vi "File et notification.vi"(8 "error in (no error)":errorcluster caption="entrée d'erreur (pas d'erreur)") -> (0 "error out":errorcluster caption="sortie d'erreur", 3 "File et Queue":T2)   [LabVIEW 2020]
uses:
  File et notification.ctl
  TypeDef/Data Event Sequenceur.ctl
  TypeDef/Liste Event Sequenceur.ctl
  TypeDef/Liste Fonction appelante.ctl
  Tache Generation Historique/Type DEF/Data Event Historique.ctl
  Tache Generation Historique/Type DEF/Liste Event Historique.ctl
  Type DEF/Commande Selection produit en cours.ctl
  TypeDef/Commande Variable Global.ctl
  Type DEF/Commande Variables Programme.ctl
  Type DEF/Commande tableau Resultat.ctl
  Instrument/BLE/Comande Variable Globale BLE.ctl
  Drivers/BLE/type_def/connection_status_bundle.ctl
  Drivers/BLE/type_def/address_type.ctl
  Type DEF/Commande Event Demande Op.ctl
  Type DEF/Commande Event Demande Autotest.ctl
  Type DEF/Commande Action Lecture RS Bridge.ctl
  Type DEF/Commande Event Saisie Op.ctl
  TypeDef/Liste fonction Saisie Operateur.ctl
  Type DEF/Commande Event Affiche Result.ctl
  Fonction/Shielding Box/Action.ctl
  TypeDef/Adresse IHM.ctl
  Commande creation.ctl
panel:
  in  "Adresse IHM":T1
  # "Application"
  # "Sequenceur"
  # "Data"
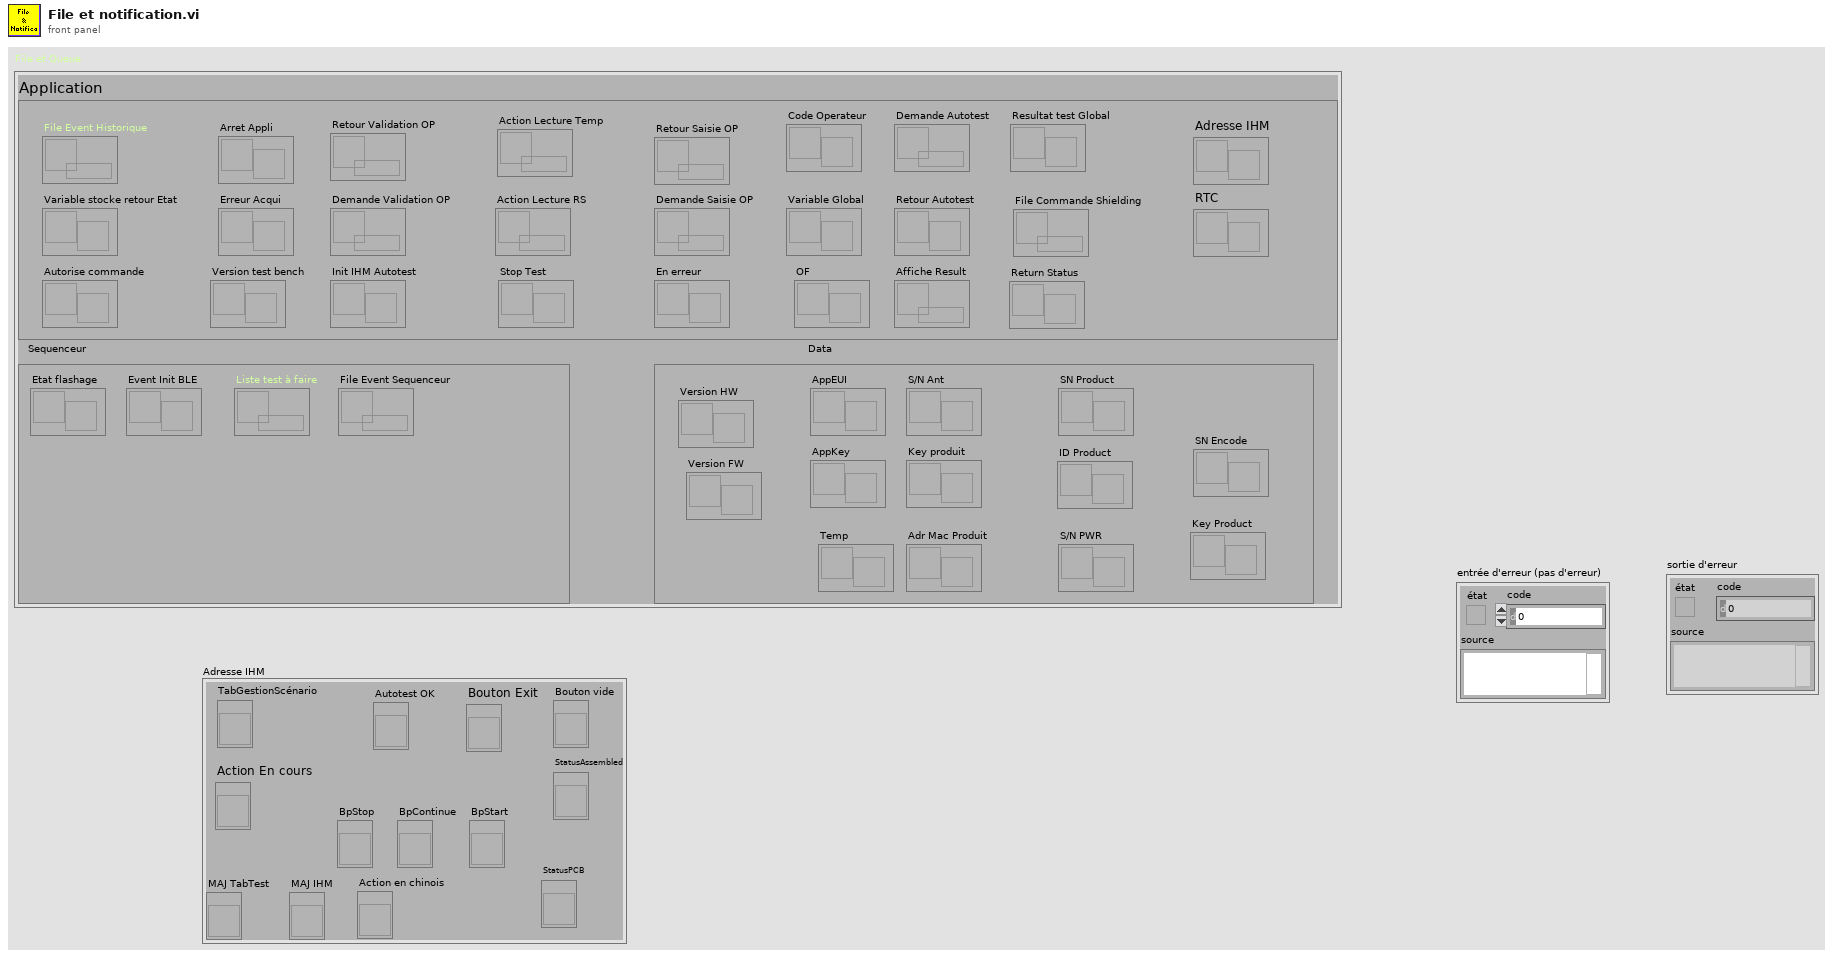
[diagram p1: front panel]
types:
  T1 = typedef "Adresse IHM.ctl" = cluster{"TabGestionScénario":refnum<vi>, "MAJ TabTest":refnum<vi>, "MAJ IHM":refnum<vi>, "BpStop":refnum<vi>, "Autotest OK":refnum<vi>, "BpContinue":refnum<vi>, "BpStart":refnum<vi>, "Action en chinois":refnum<vi>, "Bouton vide":refnum<vi>, "StatusPCB":refnum<vi>, "StatusAssembled":refnum<vi>, "Bouton Exit":refnum<vi>, "Action En cours":refnum<vi>}
  T2 = typedef "File et notification.ctl" = cluster{"Arret Appli":refnum<notifier>, "Erreur Acqui":refnum<notifier>, "File Event Sequenceur":refnum<queue>, "Liste test à faire":refnum<queue>, "File Event Historique":refnum<queue>, "Variable Global":refnum<notifier>, "Variable stocke retour Etat":refnum<notifier>, "Retour Validation OP":refnum<queue>, "Demande Validation OP":refnum<queue>, "Retour Autotest":refnum<notifier>, "Demande Autotest":refnum<queue>, "Adr Mac Produit":refnum<notifier>, "Autorise commande":refnum<notifier>, "Event Init BLE":refnum<notifier>, "Action Lecture RS":refnum<queue>, "Key produit":refnum<notifier>, "Retour Saisie OP":refnum<queue>, "Demande Saisie OP":refnum<queue>, "Etat flashage":refnum<notifier>, "Code Operateur":refnum<notifier>, "Resultat test Global":refnum<notifier>, "Stop Test":refnum<notifier>, "Init IHM Autotest":refnum<notifier>, "Version test bench":refnum<notifier>, "SN Product":refnum<notifier>, "En erreur":refnum<notifier>, "Affiche Result":refnum<queue>, "S/N PWR":refnum<notifier>, "AppEUI":refnum<notifier>, "Action Lecture Temp":refnum<queue>, "Temp":refnum<notifier>, "AppKey":refnum<notifier>, "OF":refnum<notifier>, "File Commande Shielding":refnum<queue>, "Return Status":refnum<notifier>, "ID Product":refnum<notifier>, "Version FW":refnum<notifier>, "Version HW":refnum<notifier>, "Adresse IHM":refnum<notifier>, "RTC":refnum<notifier>, "S/N Ant":refnum<notifier>, "SN Encode":refnum<notifier>, "Key Product":refnum<notifier>}
  T3 = cluster{"ExécutionScénarioPaquetCarte_TabGestionScénario":refnum<vi>, "ExécutionScénarioPaquet_TabGestionScénario":refnum<vi>, "Exécution Scénario Cigarette Panel_Panel Cigarette":refnum<vi>, "ExécutionScénarioCigarettePanel_TabGestionScénario":refnum<vi>, "ExécutionScénarioCigarette_TabGestionScénario":refnum<vi>}
  T4 = typedef "Commande creation.ctl" = enum16{"Code Operateur", "En Erreur", "Stop test en cours", "Event Sequenceur", "Resulat Test", "Liste Test Sequenceur à Faire", "Adr MAC Produit", "SN Product", "Page mem", "Key Produit", "Event Historique", "Variable Global", "Variable Stocke retour Etat", "Erreur Acquit", "Retour Validation OP", "Demande Validation OP", "Retour Saisie OP", "Demande Saisie OP", "Demande Autotest", "Retour Autotest", "Autorise commande", "Event Initialisation BLE", "Etat Flashage", "Init IHM Autotest", "Version test bench", "Affiche Result", "S/N Electronic Board", "Appkey", "AppEUI", "OF", "Shielding BOX"}
  T5 = typedef "Data Event Sequenceur.ctl" = cluster{"Data":variant, "Action":T6, "Fonction Appelante":T7, "TimeOut ou Tempo":u32, "Nb Répétition":i32, "Nom étape":string}
  T6 = typedef "Liste Event Sequenceur.ctl" = enum16{"None", "------Commun------", "Quit", "Stop", "Next Test ", "Increment state", "Command VBat", "Command 5V", "Command 24V", "Command Tension 1", "Command Tension 2", "Command Tension 3", "Stop Power Supply", "Wait Power Supply", "Msg Start-up", "Start Test", "--------Test---------", "Finish", "Enter S/N PWR", "Enter S/N ANT", "Initialization", "ID EnOcean", "ID Wirepass", "ID Wirepass By J-link", "Read Mac Address", "Test EEPROM", "Programm Software", "Programm FW", "Test LED", "Test Relay", "Test RTC", "Test Button", "Reset Factory", "Test Frequency", "Read parameter", "-------Fonction-------", "Get Manufacturer ID", "Write Key", "Read Key", "Write UID", "Read UID", "Factory Reset", "Activate Service BLE", "Factory Reset With Return", "Get device type", "Teach-In EnOcean", "Get Link Table", "Get product ID", "Learn In", "Read ID EnOcean", "Read ID Wirepass", "Read ID Wirepass By J-link", "Calibration Frequency", "Get FW version", "Get HW version", "Set HW version ANT", "Set HW version PWR", "Set S/N & HW Version", "Get Serial number", "Get mode", "Set Mode Scheduler", "Set Mode Zigbee", "Get BLE Address", "Get ZB Address", "Get RTC", "Set RTC", "Get Relay status", "Set Relay On Ch1", "Set Relay Off Ch1", "Set Relay On Ch2", "Set Relay Off Ch2", "LED Red", "LED Orange", "LED Green", "LED Off", "Read Status Button", "Read Status Switch 1", "Read Status Switch 2", "Init Ok", "-------Fonction de base-----", "Programm With J-link", "Erase All with NRF Tools", "Programm Bootloader With Commander", "Programm Erase With Commander", "Programm Applicatif With Commander", "Programm Test With Commander", "Calibration Frequency With Commander", "Init Calibration Frequency With Commander", "Encode S/N", "Creation S/N", "Save S/N", "Reset S/N", "Programm DFU", "Erase CPU", "Enable Jlink", "Disable Jlink", "Enable ICD", "Disable ICD", "Enable UART", "Disable UART", "Enable Alim Produit", "Disable Alim Produit", "Enable SW1", "Disable SW1", "Enable SW2", "Disable SW2", "Enable Multi 220V", "Disable Multi 220V", "Enable Multi V1", "Enable Multi V2", "Enable Multi V3", "Enable Multi V4", "Enable Multi V5", "Enable Multi V6", "Enable Multi V7", "Enable Multi V8", "Disable Multi", "Enable EV1", "Enable EV2", "Enable EV3", "Enable CS1", "Enable CS2", "Enable CS3", "Enable CS4", "Disable DO", "Wait Frequency", "Wait Press", "Wait Event Press", "Wait Release", "Wait Event Release", "Wait turn", "Wait Move", "Wait Remove", "Wait Power", "Waiting Back BLE", "Connect BLE", "Disconnect BLE", "Waiting Back RS", "Waiting Back SSH", "Waiting Display Operator", "Operator Input", "Operator Waiting Show", "Operator Waiting mask", "Waiting Operator", "Waiting Operator Input", "BLE Read RSSI", "Read DIO", "Read Ana 1", "Read Ana 2", "Read Ana 3", "Read Ana 4", "Read Ana 5", "Read Ana 6", "Read Ana 7", "Read Ana 8", "Write Ana 1", "Write Ana 2", "Ammeter Reading DC", "Ammeter Reading AC", "Multimeter Reading DC", "Multimeter Reading AC", "LED FEASA Reading", "Tempo 1", "Tempo 2", "Tempo 3", "Tempo 4", "Tempo 5", "Tempo 6", "Sanction", "No Sanction", "Print Label", "Write CSV", "Send Mail"}
  T7 = typedef "Liste Fonction appelante.ctl" = enum16{"None", "Open Com DUT", "Enter OF", "Serial Number", "Start-up", "Start Test", "Finish", "Enter S/N PWR", "Enter S/N ANT", "Read Mac Address", "Test Frequency", "Initialization", "ID EnOcean", "ID Wirepass", "Test Button", "Test EEPROM", "Test LED", "Test Relay", "Test RTC", "Reset Factory", "Read parameter", "Programm Software", "Programm FW", "IHM", "Print Label PCBA", "Print Label Assembled", "Print Label Packaging", "End", "Error"}
  T8 = typedef "Data Event Historique.ctl" = cluster{"Data":variant, "Event Historique":T9, "Type Carte":T10}
  T9 = typedef "Liste Event Historique.ctl" = enum16{"None", "Quit", "Ecriture Historique", "Ecriture BDD", "Send Mail", "Print Ettiquette"}
  T10 = typedef "Commande Selection produit en cours.ctl" = enum16{"None", "PCBA", "Assembled"}
  T11 = typedef "Commande Event Demande Op.ctl" = cluster{"Action":enum16{"None", "Quit", "Hidden", "Visible", "Affiche bouton", "Masque bouton"}, "Fonction Appelante":T7, "Nom etape":string, "error in (no error)":errorcluster}
  T12 = typedef "Commande Event Affiche Result.ctl" = cluster{"Action":enum16{"None", "Quit", "Hidden", "Visible"}, "Tableau élément":cluster{"Nom test":string, "Result test":bool[], "Nom pointe de test":string[], "Valeur test":string[], "Temps Etape":dbl, "Numero Etape":string[]}[], "error in (no error)":errorcluster}
  T13 = typedef "Commande Event Saisie Op.ctl" = cluster{"Action":enum16{"None", "Quit", "Hidden", "Visible", "Affiche bouton", "Masque bouton"}, "Message":string, "Txt Bouton OK":string, "Txt Bouton Nok":string, "Fonction":T14}
  T14 = typedef "Liste fonction Saisie Operateur.ctl" = enum16{"None", "Saisie S/N", "Recherche dans historique", "Recherche dans historique PCB", "Enter OF", "Enter SN PWR", "Enter SN Ant", "Validation OP"}
  T15 = typedef "Commande Event Demande Autotest.ctl" = cluster{"Action":enum16{"None", "Quit", "Hidden", "Visible", "En Cours"}, "Data":variant}
  T16 = typedef "Commande Variable Global.ctl" = cluster{"Fichier":cluster{"Chemin Save Historique":path, "Fichier Appplication":string, "Fichier Test":string, "Fichier Langue":string, "Part Number":string, "Fichier Parametre":string, "Chemin Fichier Parametre":path, "Fichier Print":string, "Fichier BDD":string}, "Liaison Serie":cluster{"RS Alimentation":refnum<visa-resource-name>, "RS Multimetre":refnum<k15>, "RS Carte":refnum<visa-resource-name>, "RS Dongle WIFI":refnum<visa-resource-name>, "RS Dongle BLE":refnum<visa-resource-name>, "RSA306":refnum<visa-resource-name>, "RS Printer PCBA":refnum<visa-resource-name>, "RS Golden Sample":refnum<visa-resource-name>, "RS Printer Ass":refnum<visa-resource-name>, "RS Printer Pack":refnum<visa-resource-name>, "RS Sonde Temp":refnum<visa-resource-name>, "RS Multimetre Bis":refnum<k15>, "RS FEASA LED":refnum<visa-resource-name>}, "Liaison DIO":cluster{"Jlink":cluster{"Line":tag, "Nom Voie":string, "Nom device in INI":string}[], "ICD":cluster{"Line":tag, "Nom Voie":string, "Nom device in INI":string}[], "UART":cluster{"Line":tag, "Nom Voie":string, "Nom device in INI":string}[], "Multi1":cluster{"Line":tag, "Nom Voie":string, "Nom device in INI":string}[], "Multi2":cluster{"Line":tag, "Nom Voie":string, "Nom device in INI":string}[], "Multi3":cluster{"Line":tag, "Nom Voie":string, "Nom device in INI":string}[], "DO1":cluster{"Line":tag, "Nom Voie":string, "Nom device in INI":string}[], "DO2":cluster{"Line":tag, "Nom Voie":string, "Nom device in INI":string}[], "DO3":cluster{"Line":tag, "Nom Voie":string, "Nom device in INI":string}[], "AlimProduct":cluster{"Line":tag, "Nom Voie":string, "Nom device in INI":string}[], "SW2":cluster{"Line":tag, "Nom Voie":string, "Nom device in INI":string}[], "SW1":cluster{"Line":tag, "Nom Voie":string, "Nom device in INI":string}[], "Multi220V_CPT":cluster{"Line":tag, "Nom Voie":string, "Nom device in INI":string}[]}, "Variable Programme":T17, "Information Entete":cluster{"Opérateur":string, "Ordre de fabrication":string, "Numéro de lot":string, "Commentaire":string}, "Nom de périphérique DAQmx":tag, "Parameter RF":cluster{"Frequency CW":string, "FrequencyRX":string, "TimeOutRX":string}, "Divers":cluster{"DUT Hub":u32}, "Analogique":cluster{"AI1":cluster{"Voie":tag, "Nom Voie":string, "Nom device in INI":string}[], "Ai2":cluster{"Voie":tag, "Nom Voie":string, "Nom device in INI":string}[], "AI3":cluster{"Voie":tag, "Nom Voie":string, "Nom device in INI":string}[], "AI4":cluster{"Voie":tag, "Nom Voie":string, "Nom device in INI":string}[], "AI5":cluster{"Voie":tag, "Nom Voie":string, "Nom device in INI":string}[], "AI6":cluster{"Voie":tag, "Nom Voie":string, "Nom device in INI":string}[], "AI7":cluster{"Voie":tag, "Nom Voie":string, "Nom device in INI":string}[], "AI8":cluster{"Voie":tag, "Nom Voie":string, "Nom device in INI":string}[], "AO1":cluster{"Voie":tag, "Nom Voie":string, "Nom device in INI":string}[], "AO2":cluster{"Voie":tag, "Nom Voie":string, "Nom device in INI":string}[]}, "Parametre BLE":T19, "Shielding Box":cluster{"Comm":refnum<visa-resource-name>, "Used":bool}, "Challenge Bit":u8[]}
  T17 = typedef "Commande Variables Programme.ctl" = cluster{"Cigarette en cours":i32, "Tableau Resultat test":T18, "Test en cours":i32, "Type test":string, "Type Carte":T10, "Test Select":cluster{"Booléen 4":bool}[]}
  T18 = typedef "Commande tableau Resultat.ctl" = cluster{"Resultat produit":cluster{"Nom test":string, "Result test":bool[], "Nom pointe de test":string[], "Valeur test":string[], "Temps Etape":dbl, "Numero Etape":string[]}[]}[]
  T19 = typedef "Comande Variable Globale BLE.ctl" = cluster{"Devices Connect":string[][], "Connection Status":T20, "Handle table":string[][], "Service":string, "characteristic Read":string, "characteristic Write":string, "Port BLE":refnum<visa-resource-name>, "Nb Packet Light":u8}
  T20 = typedef "connection_status_bundle.ctl" = cluster{"MAC Address":string, "cnx handle":u8, "cnx flags":u8, "Address Type":T21, "Connection Interval (ms)":u16, "Timeout(ms)":u16, "Latency":u16, "bonding handle":u8}
  T21 = typedef "address_type.ctl" = u8
  T22 = typedef "Action.ctl" = enum16{"Open Shielding", "Close Shielding", "Read Status", "Stop Wait Start", "Wait Start", "Wait Close", "Wait Open", "Quit"}
  T23 = cluster{"[0]":refnum<notifier>, "[1]":refnum<notifier>, "[2]":refnum<notifier>, "[3]":refnum<notifier>, "[4]":refnum<notifier>, "[5]":refnum<notifier>}
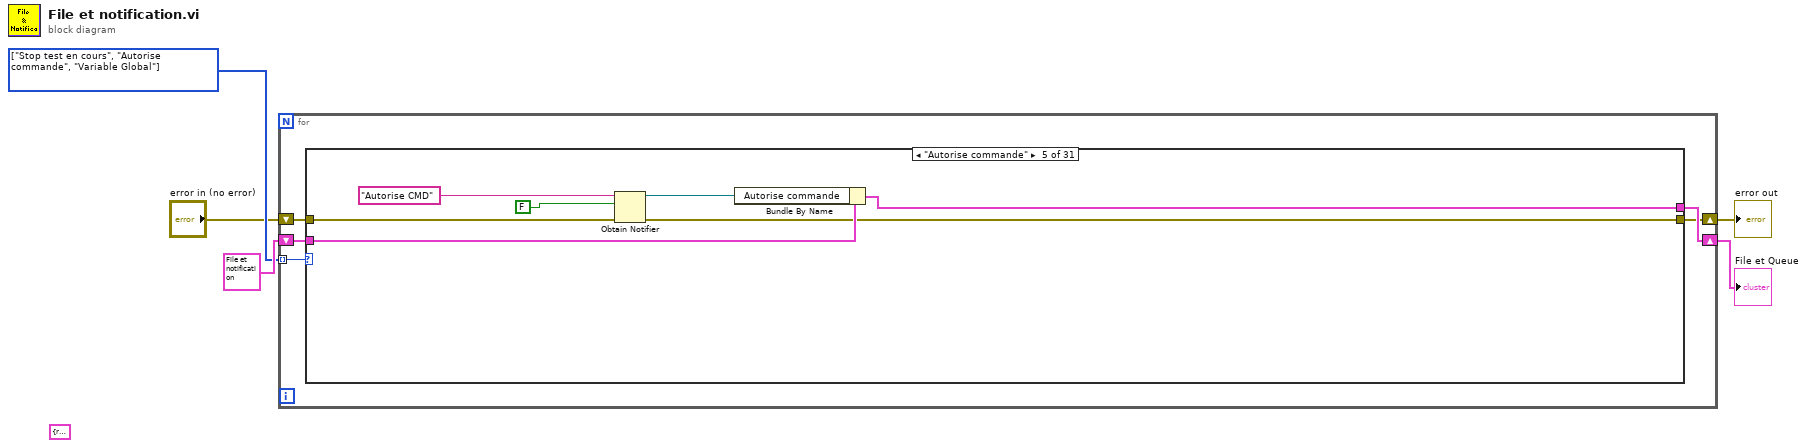
[diagram p0: block diagram]
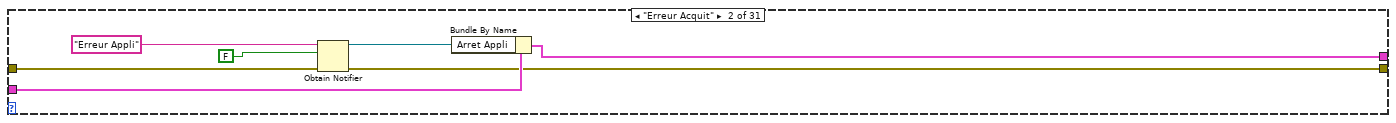
[diagram p3: hidden frame]
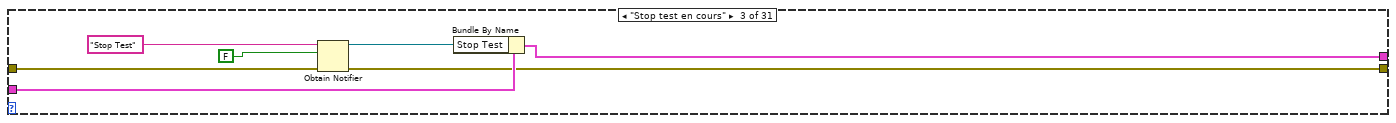
[diagram p4: hidden frame]
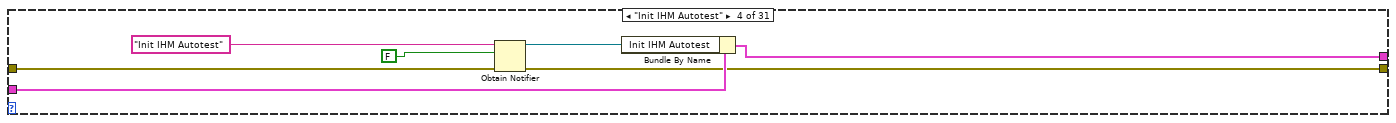
[diagram p5: hidden frame]
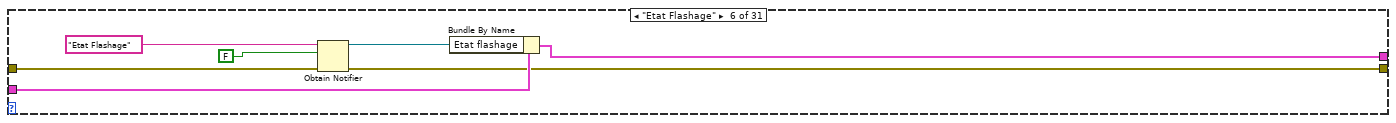
[diagram p6: hidden frame]
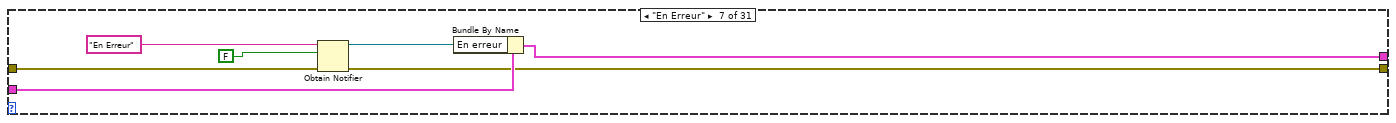
[diagram p7: hidden frame]
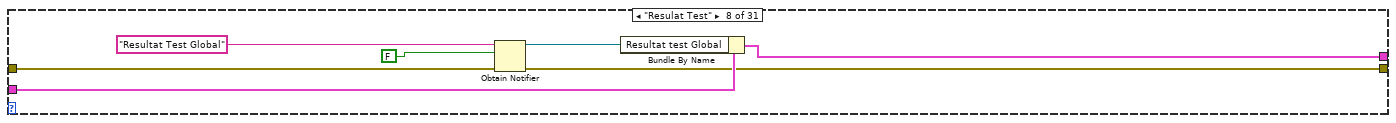
[diagram p8: hidden frame]
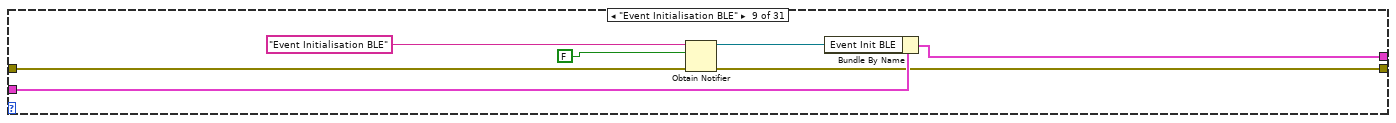
[diagram p9: hidden frame]
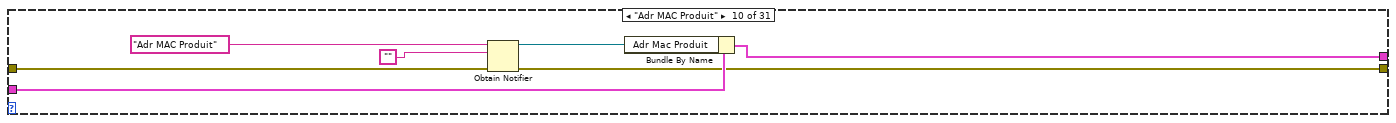
[diagram p10: hidden frame]
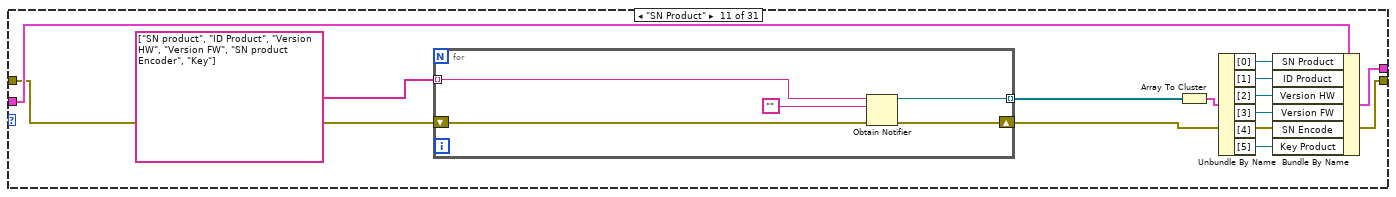
[diagram p11: hidden frame]
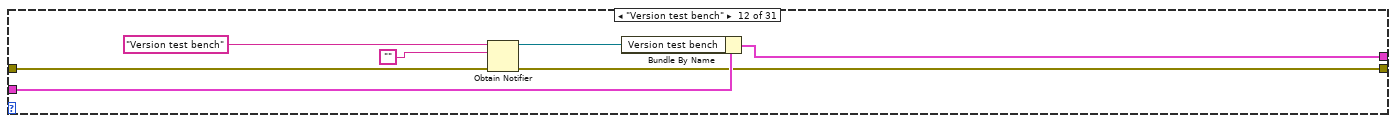
[diagram p12: hidden frame]
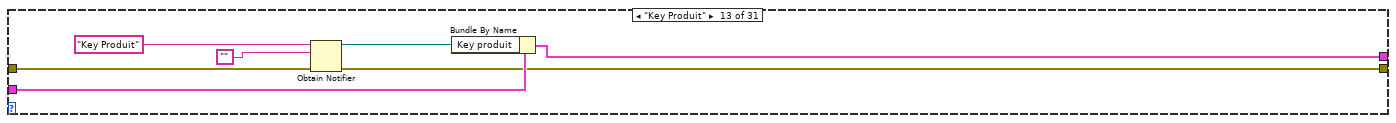
[diagram p13: hidden frame]
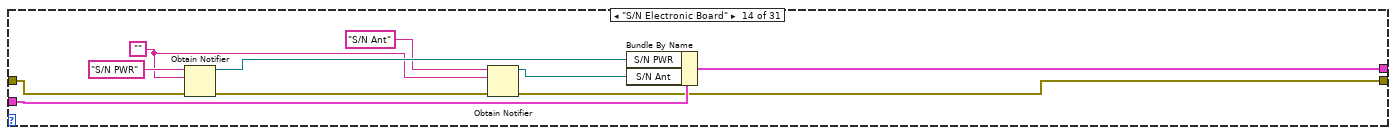
[diagram p14: hidden frame]
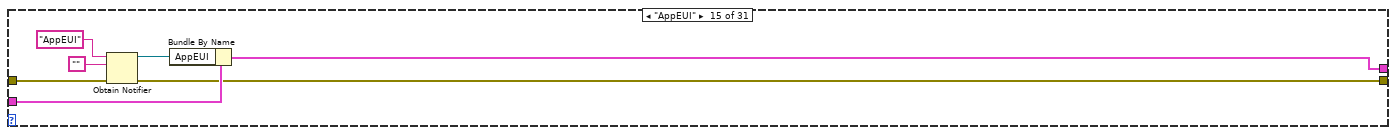
[diagram p15: hidden frame]
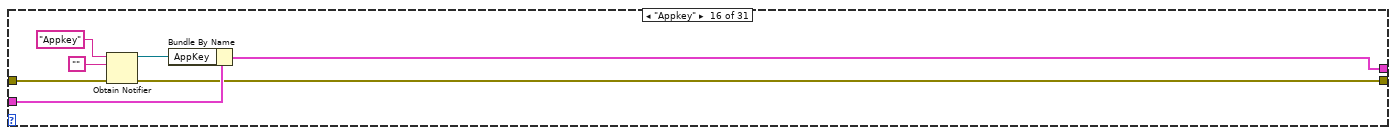
[diagram p16: hidden frame]
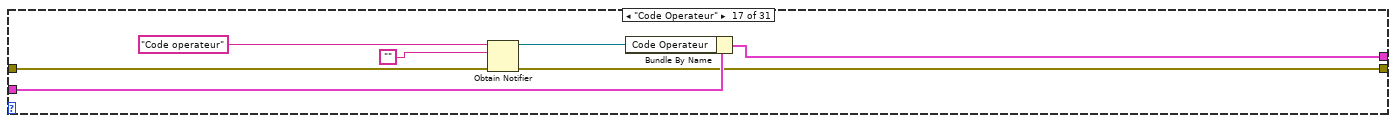
[diagram p17: hidden frame]
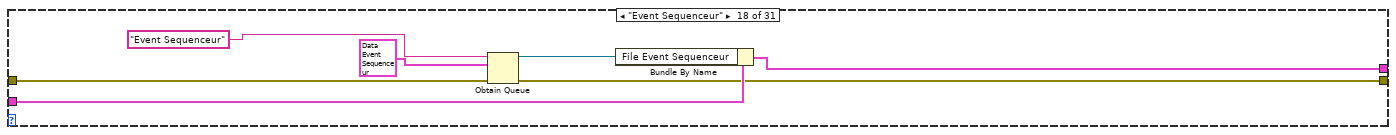
[diagram p18: hidden frame]
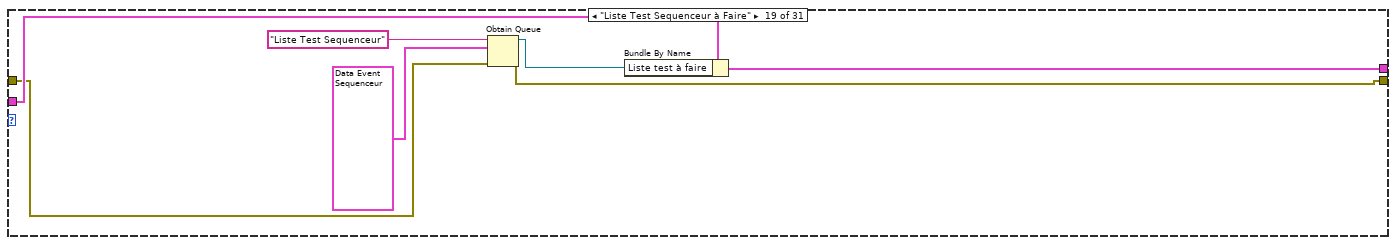
[diagram p19: hidden frame]
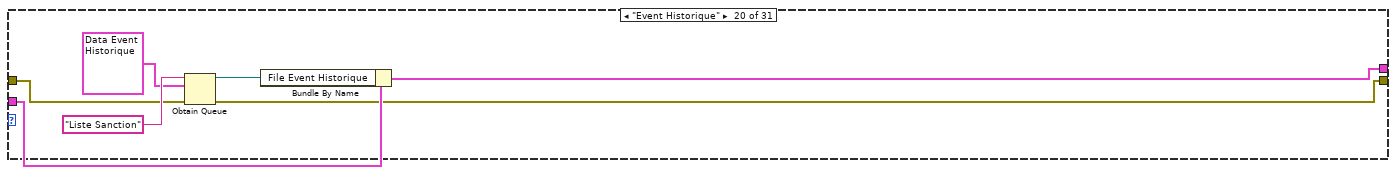
[diagram p20: hidden frame]
diagram:
  (unwired) T3 {"ExécutionScénarioPaquetCarte_TabGestionScénario"=refnum, "ExécutionScénarioPaquet_TabGestionScénario"=refnum, "Exécution Scénario Cigarette Panel_Panel Cigarette"=refnum, "ExécutionScénarioCigarettePanel_TabGestionScénario"=refnum, "ExécutionScénarioCigarette_TabGestionScénario"=refnum} ("Cluster")
  w4 = T4[] [enum."Stop test en cours", enum."Autorise commande", enum."Variable Global"] items=["Code Operateur", "En Erreur", "Stop test en cours", "Event Sequenceur", "Resulat Test", "Liste Test Sequenceur à Faire", "Adr MAC Produit", "SN Product", "Page mem", "Key Produit", "Event Historique", "Variable Global", "Variable Stocke retour Etat", "Erreur Acquit", "Retour Validation OP", "Demande Validation OP", "Retour Saisie OP", "Demande Saisie OP", "Demande Autotest", "Retour Autotest", "Autorise commande", "Event Initialisation BLE", "Etat Flashage", "Init IHM Autotest", "Version test bench", "Affiche Result", "S/N Electronic Board", "Appkey", "AppEUI", "OF", "Shielding BOX"]
  n1 = for {
    tunnel: w4 -> [w10] mode=indexing
    shift-right: [w8] -> w3
    shift-left: T2 {"Arret Appli"=refnum, "Erreur Acqui"=refnum, "File Event Sequenceur"=refnum, "Liste test à faire"=refnum, "File Event Historique"=refnum, "Variable Global"=refnum, "Variable stocke retour Etat"=refnum, "Retour Validation OP"=refnum, "Demande Validation OP"=refnum, "Retour Autotest"=refnum, "Demande Autotest"=refnum, "Adr Mac Produit"=refnum, "Autorise commande"=refnum, "Event Init BLE"=refnum, "Action Lecture RS"=refnum, "Key produit"=refnum, "Retour Saisie OP"=refnum, "Demande Saisie OP"=refnum, "Etat flashage"=refnum, "Code Operateur"=refnum, "Resultat test Global"=refnum, "Stop Test"=refnum, "Init IHM Autotest"=refnum, "Version test bench"=refnum, "SN Product"=refnum, "En erreur"=refnum, "Affiche Result"=refnum, "S/N PWR"=refnum, "AppEUI"=refnum, "Action Lecture Temp"=refnum, "Temp"=refnum, "AppKey"=refnum, "OF"=refnum, "File Commande Shielding"=refnum, "Return Status"=refnum, "ID Product"=refnum, "Version FW"=refnum, "Version HW"=refnum, "Adresse IHM"=refnum, "RTC"=refnum, "S/N Ant"=refnum, "SN Encode"=refnum, "Key Product"=refnum} -> [w9]
    shift-right: [w6] -> w1
    shift-left: "error in (no error)" -> [w7]
    n2 = case shown="\"Autorise commande\"" w10 {
      tunnel: w9 -> [w11 w17 w24 w31 w38 w45 w52 w59 w66 w74 w88 w99 w106 w116 w123 w130 w137 w144 w151 w158 w165 w172 w179 w186 w201 w208 w217 w224 w231 w233 w243]
      tunnel: [w11 w15 w22 w29 w36 w43 w50 w57 w64 w73 w87 w98 w105 w115 w122 w129 w136 w143 w150 w157 w164 w171 w178 w185 w200 w207 w216 w223 w230 w234 w242] -> w8
      tunnel: w7 -> [w12 w14 w21 w28 w35 w42 w49 w55 w63 w72 w86 w97 w104 w114 w121 w128 w135 w142 w149 w156 w163 w170 w177 w184 w196 w206 w215 w222 w229 w236 w244]
      tunnel: [w12 w13 w20 w27 w34 w41 w48 w56 w62 w71 w85 w96 w103 w111 w120 w127 w134 w141 w148 w155 w162 w169 w174 w183 w199 w205 w212 w221 w228 w235 w241] -> w6
      frame Default {
      }
      frame "Erreur Acquit" {
        n3 = Obtain Notifier(name (unnamed)="Erreur Appli" ("nom (aucun)"), notification data type=FALSE, error in (no error)=w14) -> (notifier out=w16:refnum<notifier>, error out=w13:errorcluster)  [unwired: 1 in, 1 out]
        n4 = Bundle By Name(cluster=w17, "Arret Appli"=w16) -> (w15:T2)
      }
      frame "Stop test en cours" {
        n5 = Obtain Notifier(name (unnamed)="Stop Test" ("nom (aucun)"), notification data type=FALSE, error in (no error)=w21) -> (notifier out=w23:refnum<notifier>, error out=w20:errorcluster)  [unwired: 1 in, 1 out]
        n6 = Bundle By Name(cluster=w24, "Stop Test"=w23) -> (w22:T2)
      }
      frame "Init IHM Autotest" {
        n7 = Obtain Notifier(name (unnamed)="Init IHM Autotest" ("nom (aucun)"), notification data type=FALSE, error in (no error)=w28) -> (notifier out=w30:refnum<notifier>, error out=w27:errorcluster)  [unwired: 1 in, 1 out]
        n8 = Bundle By Name(cluster=w31, "Init IHM Autotest"=w30) -> (w29:T2)
      }
      frame "Autorise commande" {
        n9 = Obtain Notifier(name (unnamed)="Autorise CMD" ("nom (aucun)"), notification data type=FALSE, error in (no error)=w35) -> (notifier out=w37:refnum<notifier>, error out=w34:errorcluster)  [unwired: 1 in, 1 out]
        n10 = Bundle By Name(cluster=w38, "Autorise commande"=w37) -> (w36:T2)
      }
      frame "Etat Flashage" {
        n11 = Obtain Notifier(name (unnamed)="Etat Flashage" ("nom (aucun)"), notification data type=FALSE, error in (no error)=w42) -> (notifier out=w44:refnum<notifier>, error out=w41:errorcluster)  [unwired: 1 in, 1 out]
        n12 = Bundle By Name(cluster=w45, "Etat flashage"=w44) -> (w43:T2)
      }
      frame "En Erreur" {
        n13 = Obtain Notifier(name (unnamed)="En Erreur" ("nom (aucun)"), notification data type=FALSE, error in (no error)=w49) -> (notifier out=w51:refnum<notifier>, error out=w48:errorcluster)  [unwired: 1 in, 1 out]
        n14 = Bundle By Name(cluster=w52, "En erreur"=w51) -> (w50:T2)
      }
      frame "Resulat Test" {
        n15 = Obtain Notifier(name (unnamed)="Resultat Test Global" ("nom (aucun)"), notification data type=FALSE, error in (no error)=w55) -> (notifier out=w58:refnum<notifier>, error out=w56:errorcluster)  [unwired: 1 in, 1 out]
        n16 = Bundle By Name(cluster=w59, "Resultat test Global"=w58) -> (w57:T2)
      }
      frame "Event Initialisation BLE" {
        n17 = Obtain Notifier(name (unnamed)="Event Initialisation BLE" ("nom (aucun)"), notification data type=FALSE, error in (no error)=w63) -> (notifier out=w65:refnum<notifier>, error out=w62:errorcluster)  [unwired: 1 in, 1 out]
        n18 = Bundle By Name(cluster=w66, "Event Init BLE"=w65) -> (w64:T2)
      }
      frame "Adr MAC Produit" {
        n19 = Obtain Notifier(name (unnamed)="Adr MAC Produit" ("nom (aucun)"), notification data type="", error in (no error)=w72) -> (notifier out=w69:refnum<notifier>, error out=w71:errorcluster)  [unwired: 1 in, 1 out]
        n20 = Bundle By Name(cluster=w74, "Adr Mac Produit"=w69) -> (w73:T2)
      }
      frame "SN Product" {
        n21 = for {
          shift-right: [w92] -> w85
          shift-left: w86 -> [w93]
          tunnel: string[] ["SN product", "ID Product", "Version HW", "Version FW", "SN product Encoder", "Key"] -> [w90] mode=indexing
          tunnel: [w89] -> w83 mode=indexing
          n22 = Obtain Notifier(name (unnamed)=w90, notification data type="", error in (no error)=w93) -> (notifier out=w89:refnum<notifier>, error out=w92:errorcluster)  [unwired: 1 in, 1 out]
        }
        n23 = Array To Cluster(array=w83) -> (cluster=w82:T23)
        n24 = Unbundle By Name(w82) -> ("[0]"=w81:refnum<notifier>, "[1]"=w80:refnum<notifier>, "[2]"=w79:refnum<notifier>, "[3]"=w78:refnum<notifier>, "[4]"=w77:refnum<notifier>, "[5]"=w76:refnum<notifier>)
        n25 = Bundle By Name(cluster=w88, "SN Product"=w81, "ID Product"=w80, "Version HW"=w79, "Version FW"=w78, "SN Encode"=w77, "Key Product"=w76) -> (w87:T2)
      }
      frame "Version test bench" {
        n26 = Obtain Notifier(name (unnamed)="Version test bench" ("nom (aucun)"), notification data type="", error in (no error)=w97) -> (notifier out=w94:refnum<notifier>, error out=w96:errorcluster)  [unwired: 1 in, 1 out]
        n27 = Bundle By Name(cluster=w99, "Version test bench"=w94) -> (w98:T2)
      }
      frame "Key Produit" {
        n28 = Obtain Notifier(name (unnamed)="Key Produit" ("nom (aucun)"), notification data type="", error in (no error)=w104) -> (notifier out=w101:refnum<notifier>, error out=w103:errorcluster)  [unwired: 1 in, 1 out]
        n29 = Bundle By Name(cluster=w106, "Key produit"=w101) -> (w105:T2)
      }
      frame "S/N Electronic Board" {
        w109 = ""
        n30 = Obtain Notifier(name (unnamed)="S/N PWR" ("nom (aucun)"), notification data type=w109, error in (no error)=w114) -> (notifier out=w113:refnum<notifier>, error out=w112:errorcluster)  [unwired: 1 in, 1 out]
        n31 = Obtain Notifier(name (unnamed)="S/N Ant" ("nom (aucun)"), notification data type=w109, error in (no error)=w112) -> (notifier out=w108:refnum<notifier>, error out=w111:errorcluster)  [unwired: 1 in, 1 out]
        n32 = Bundle By Name(cluster=w116, "S/N PWR"=w113, "S/N Ant"=w108) -> (w115:T2)
      }
      frame "AppEUI" {
        n33 = Obtain Notifier(name (unnamed)="AppEUI" ("nom (aucun)"), notification data type="", error in (no error)=w121) -> (notifier out=w118:refnum<notifier>, error out=w120:errorcluster)  [unwired: 1 in, 1 out]
        n34 = Bundle By Name(cluster=w123, "AppEUI"=w118) -> (w122:T2)
      }
      frame "Appkey" {
        n35 = Obtain Notifier(name (unnamed)="Appkey" ("nom (aucun)"), notification data type="", error in (no error)=w128) -> (notifier out=w125:refnum<notifier>, error out=w127:errorcluster)  [unwired: 1 in, 1 out]
        n36 = Bundle By Name(cluster=w130, "AppKey"=w125) -> (w129:T2)
      }
      frame "Code Operateur" {
        n37 = Obtain Notifier(name (unnamed)="Code operateur" ("nom (aucun)"), notification data type="", error in (no error)=w135) -> (notifier out=w132:refnum<notifier>, error out=w134:errorcluster)  [unwired: 1 in, 1 out]
        n38 = Bundle By Name(cluster=w137, "Code Operateur"=w132) -> (w136:T2)
      }
      frame "Event Sequenceur" {
        n39 = Obtain Queue(name (unnamed)="Event Sequenceur" ("nom (aucun)"), element data type=T5 {"Data"=variant, "Action"=enum."None", "Fonction Appelante"=enum."None", "TimeOut ou Tempo"=0, "Nb Répétition"=0, "Nom étape"=""} ("Data Event Séquenceur"), error in (no error)=w142) -> (queue out=w139:refnum<queue>, error out=w141:errorcluster)  [unwired: 2 in, 1 out]
        n40 = Bundle By Name(cluster=w144, "File Event Sequenceur"=w139) -> (w143:T2)
      }
      frame "Liste Test Sequenceur à Faire" {
        n41 = Obtain Queue(name (unnamed)="Liste Test Sequenceur" ("nom (aucun)"), element data type=T5 {"Data"=variant, "Action"=enum."None", "Fonction Appelante"=enum."None", "TimeOut ou Tempo"=0, "Nb Répétition"=0, "Nom étape"=""} ("Data Event Séquenceur"), error in (no error)=w149) -> (queue out=w146:refnum<queue>, error out=w148:errorcluster)  [unwired: 2 in, 1 out]
        n42 = Bundle By Name(cluster=w151, "Liste test à faire"=w146) -> (w150:T2)
      }
      frame "Event Historique" {
        n43 = Obtain Queue(name (unnamed)="Liste Sanction" ("nom (aucun)"), element data type=T8 {"Data"=variant, "Event Historique"=enum."None", "Type Carte"=enum."None"} ("Data Event Séquenceur"), error in (no error)=w156) -> (queue out=w153:refnum<queue>, error out=w155:errorcluster)  [unwired: 2 in, 1 out]
        n44 = Bundle By Name(cluster=w158, "File Event Historique"=w153) -> (w157:T2)
      }
      frame "Demande Validation OP" {
        n45 = Obtain Queue(name (unnamed)="Demande Validattion OP" ("nom (aucun)"), element data type=T11 {"Action"=enum."Visible", "Fonction Appelante"=enum."None", "Nom etape"="", "error in (no error)"={"status"=FALSE, "code"=0, "source"=""}}, error in (no error)=w163) -> (queue out=w160:refnum<queue>, error out=w162:errorcluster)  [unwired: 2 in, 1 out]
        n46 = Bundle By Name(cluster=w165, "Demande Validation OP"=w160) -> (w164:T2)
      }
      frame "Affiche Result" {
        n47 = Obtain Queue(name (unnamed)="Affiche result" ("nom (aucun)"), element data type=T12 {"Action"=enum."Visible", "Tableau élément"=[], "error in (no error)"={"status"=FALSE, "code"=0, "source"=""}}, error in (no error)=w170) -> (queue out=w167:refnum<queue>, error out=w169:errorcluster)  [unwired: 2 in, 1 out]
        n48 = Bundle By Name(cluster=w172, "Affiche Result"=w167) -> (w171:T2)
      }
      frame "Demande Saisie OP" {
        n49 = Obtain Queue(name (unnamed)="Demande Saisie OP" ("nom (aucun)"), element data type=T13 {"Action"=enum."Visible", "Message"="", "Txt Bouton OK"="", "Txt Bouton Nok"="", "Fonction"=enum."None"}, error in (no error)=w177) -> (queue out=w176:refnum<queue>, error out=w174:errorcluster)  [unwired: 2 in, 1 out]
        n50 = Bundle By Name(cluster=w179, "Demande Saisie OP"=w176) -> (w178:T2)
      }
      frame "Demande Autotest" {
        n51 = Obtain Queue(name (unnamed)="Demande Autotest" ("nom (aucun)"), element data type=T15 {"Action"=enum."Visible", "Data"=variant(string "")}, error in (no error)=w184) -> (queue out=w181:refnum<queue>, error out=w183:errorcluster)  [unwired: 2 in, 1 out]
        n52 = Bundle By Name(cluster=w186, "Demande Autotest"=w181) -> (w185:T2)
      }
      frame "Variable Global" {
        n53 = Obtain Notifier(name (unnamed)="Adresse IHM" ("nom (aucun)"), notification data type="Adresse IHM", error in (no error)=w196) -> (notifier out=w188:refnum<notifier>, error out=w193:errorcluster)  [unwired: 1 in, 1 out]
        n54 = Obtain Notifier(name (unnamed)="RTC" ("nom (aucun)"), notification data type=timestamp(0 s since 1904-01-01), error in (no error)=w193) -> (notifier out=w189:refnum<notifier>, error out=w190:errorcluster)  [unwired: 1 in, 1 out]
        n55 = Obtain Notifier(name (unnamed)="Variable Gobal" ("nom (aucun)"), notification data type=T16 {"Fichier"={"Chemin Save Historique"=path "", "Fichier Appplication"="", "Fichier Test"="", "Fichier Langue"="", "Part Number"="", "Fichier Parametre"="", "Chemin Fichier Parametre"=path "", "Fichier Print"="", "Fichier BDD"=""}, "Liaison Serie"={"RS Alimentation"="", "RS Multimetre"="", "RS Carte"="", "RS Dongle WIFI"="", "RS Dongle BLE"="", "RSA306"="", "RS Printer PCBA"="", "RS Golden Sample"="", "RS Printer Ass"="", "RS Printer Pack"="", "RS Sonde Temp"="", "RS Multimetre Bis"="", "RS FEASA LED"=""}, "Liaison DIO"={"Jlink"=[], "ICD"=[], "UART"=[], "Multi1"=[], "Multi2"=[], "Multi3"=[], "DO1"=[], "DO2"=[], "DO3"=[], "AlimProduct"=[], "SW2"=[], "SW1"=[], "Multi220V_CPT"=[]}, "Variable Programme"={"Cigarette en cours"=0, "Tableau Resultat test"=[], "Test en cours"=0, "Type test"="", "Type Carte"=enum."None", "Test Select"=[]}, "Information Entete"={"Opérateur"="", "Ordre de fabrication"="", "Numéro de lot"="", "Commentaire"=""}, "Nom de périphérique DAQmx"="", "Parameter RF"={"Frequency CW"="", "FrequencyRX"="", "TimeOutRX"=""}, "Divers"={"DUT Hub"=0}, "Analogique"={"AI1"=[], "Ai2"=[], "AI3"=[], "AI4"=[], "AI5"=[], "AI6"=[], "AI7"=[], "AI8"=[], "AO1"=[], "AO2"=[]}, "Parametre BLE"={"Devices Connect"=[], "Connection Status"={"MAC Address"="", "cnx handle"=0, "cnx flags"=0, "Address Type"=0, "Connection Interval (ms)"=0, "Timeout(ms)"=0, "Latency"=0, "bonding handle"=0}, "Handle table"=[], "Service"="", "characteristic Read"="", "characteristic Write"="", "Port BLE"="", "Nb Packet Light"=0}, "Shielding Box"={"Comm"="", "Used"=FALSE}, "Challenge Bit"=[]} ("Cluster"), error in (no error)=w190) -> (notifier out=w197:refnum<notifier>, error out=w199:errorcluster)  [unwired: 1 in, 1 out]
        n56 = Bundle By Name(cluster=w201, "Variable Global"=w197, "Adresse IHM"=w188, "RTC"=w189) -> (w200:T2)
      }
      frame "Retour Validation OP" {
        n57 = Obtain Queue(name (unnamed)="Retour Validation OP" ("nom (aucun)"), element data type=FALSE, error in (no error)=w206) -> (queue out=w203:refnum<queue>, error out=w205:errorcluster)  [unwired: 2 in, 1 out]
        n58 = Bundle By Name(cluster=w208, "Retour Validation OP"=w203) -> (w207:T2)
      }
      frame "Retour Saisie OP" {
        w211 = cluster{"Continuer":bool, "Saisie":string} {"Continuer"=FALSE, "Saisie"=""}
        n59 = Obtain Queue(name (unnamed)="Retour Saisie OP" ("nom (aucun)"), element data type=w211, error in (no error)=w215) -> (queue out=w214:refnum<queue>, error out=w213:errorcluster)  [unwired: 2 in, 1 out]
        n60 = Bundle By Name(cluster=w217, "Retour Saisie OP"=w214) -> (w216:T2)
        n61 = Obtain Queue(name (unnamed)="Retour Saisie OP Packaging" ("nom (aucun)"), element data type=w211, error in (no error)=w213) -> (error out=w212:errorcluster)  [unwired: 2 in, 2 out]
      }
      frame "Retour Autotest" {
        n62 = Obtain Notifier(name (unnamed)="Retour Autotest" ("nom (aucun)"), notification data type=FALSE, error in (no error)=w222) -> (notifier out=w219:refnum<notifier>, error out=w221:errorcluster)  [unwired: 1 in, 1 out]
        n63 = Bundle By Name(cluster=w224, "Retour Autotest"=w219) -> (w223:T2)
      }
      frame "Variable Stocke retour Etat" {
        n64 = Obtain Notifier(name (unnamed)="Variable Stocke retour Etat" ("nom (aucun)"), notification data type=cluster{"Retour Etat":string[], "Erreur":bool} {"Retour Etat"=[], "Erreur"=TRUE}, error in (no error)=w229) -> (notifier out=w226:refnum<notifier>, error out=w228:errorcluster)  [unwired: 1 in, 1 out]
        n65 = Bundle By Name(cluster=w231, "Variable stocke retour Etat"=w226) -> (w230:T2)
      }
      frame "OF" {
        n66 = Obtain Notifier(name (unnamed)="OF" ("nom (aucun)"), notification data type="", error in (no error)=w236) -> (notifier out=w237:refnum<notifier>, error out=w235:errorcluster)  [unwired: 1 in, 1 out]
        n67 = Bundle By Name(cluster=w233, "OF"=w237) -> (w234:T2)
      }
      frame "Shielding BOX" {
        n68 = Obtain Queue(name (unnamed)="File Commande Shielding" ("nom (aucun)"), element data type=Action."Wait Start", error in (no error)=w244) -> (queue out=w240:refnum<queue>, error out=w246:errorcluster)  [unwired: 2 in, 1 out]
        n69 = Obtain Notifier(name (unnamed)="Return Status" ("nom (aucun)"), notification data type="", error in (no error)=w246) -> (notifier out=w245:refnum<notifier>, error out=w241:errorcluster)  [unwired: 1 in, 1 out]
        n70 = Bundle By Name(cluster=w243, "File Commande Shielding"=w240, "Return Status"=w245) -> (w242:T2)
      }
    }
  }
  "File et Queue" <- w3
  "error out" <- w1
